vi "TCP_comms_test_receive.vi"() -> ()   [LabVIEW 2018]
panel:
  out "connection ID":refnum<k5>
  in  "Open Connection":bool
  in  "address":string="192.168.0.34"
  out "Received value/i":u32
  out "Connection opened?":bool
  out "Error Out":errorcluster
  in  "Stop and Exit":bool
  in  "Error In":errorcluster
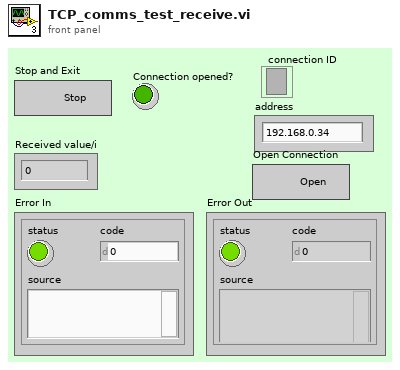
[diagram p1: front panel]
types:
  T1 = enum16{"Standard", "Buffered", "CRLF", "Immediate"}
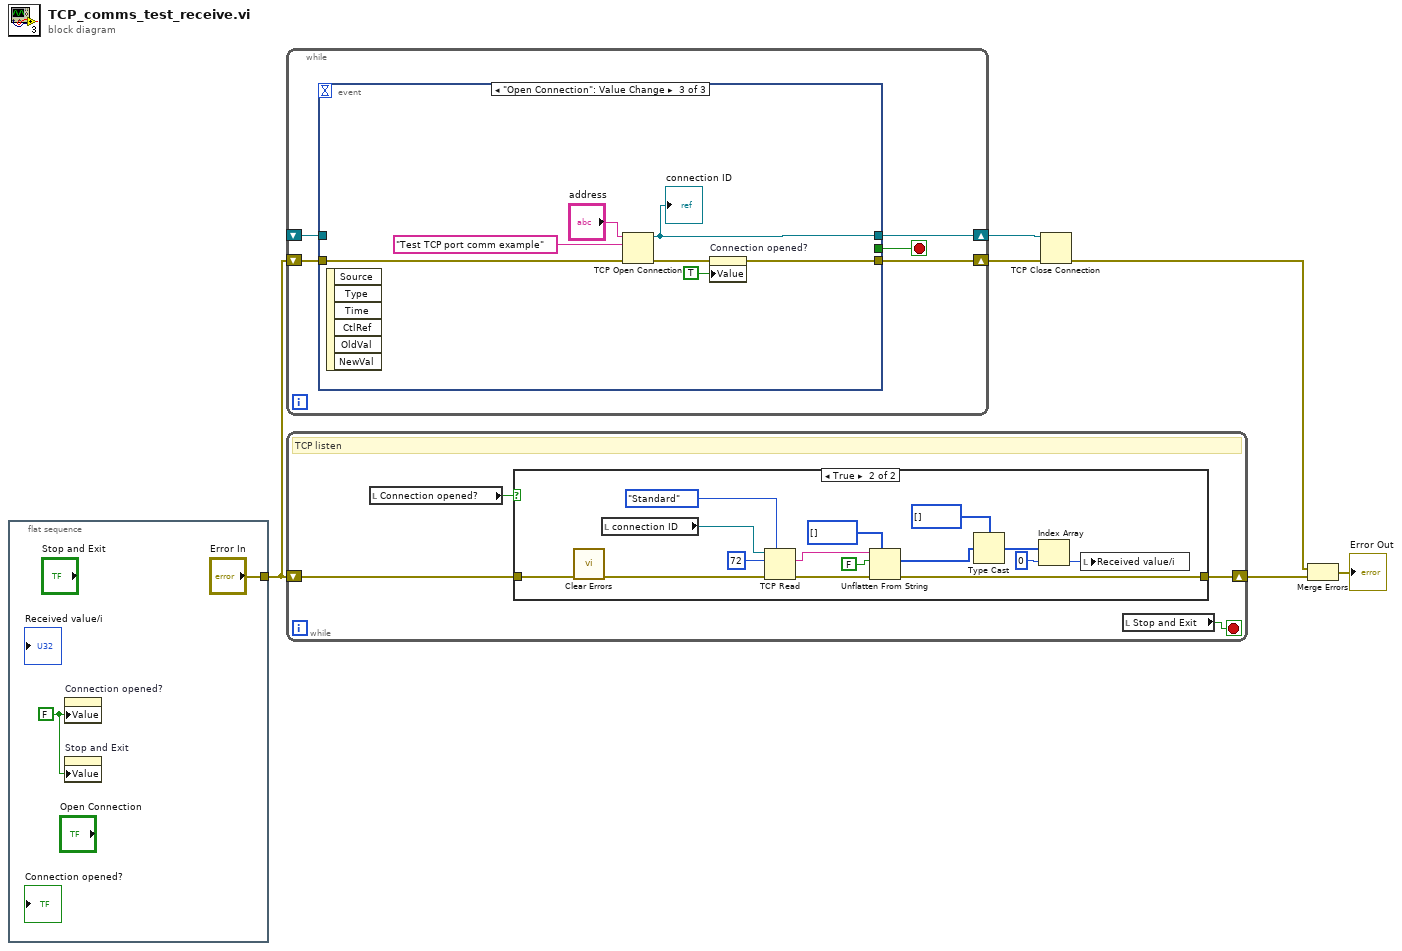
[diagram p0: block diagram]
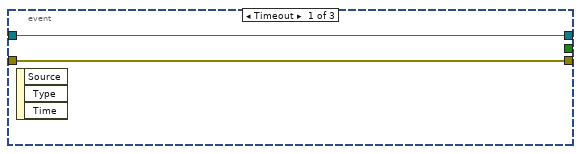
[diagram p3: hidden frame]
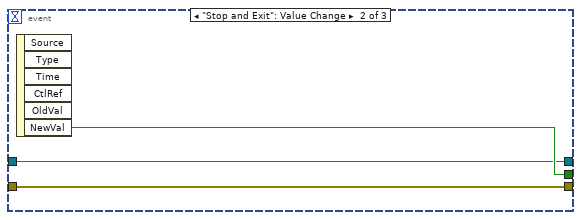
[diagram p4: hidden frame]
diagram:
  n1 = flat-sequence {
    tunnel: ["Error In"] -> w6
    frame #0 {
      w7 = FALSE ("Stop and Exit")
      n2 = property on="Connection opened?" class="Bool (strict)"("Value"=w7) -> ()  [unwired: 2 in, 2 out]
      n3 = property on="Stop and Exit" class="Bool (strict)"("Value"=w7) -> ()  [unwired: 2 in, 2 out]
    }
  }
  n4 = while {
    shift-right: [w11] -> w4
    shift-left: w6 -> [w12]
    shift-right: [w10] -> w1
    shift-left: _ -> [w9]
    stop <- w13 stop-if-true
    n5 = event shown="[2] \"Open Connection\": Value Change" {
      selector: _ -> [_ _ _]
      dyn-events: _ -> [_ _ _]
      timeout: _ -> [_ _ _]
      tunnel: [_ w18 _] -> w13
      tunnel: w12 -> [w15 w17 w25]
      tunnel: [w15 w17 w21] -> w11
      tunnel: [w14 w16 w19] -> w10
      tunnel: w9 -> [w14 w16 _]
      event Timeout {
        n6 = event-data() -> ()  [unwired: 1 in, 3 out]
      }
      event "Stop and Exit": Value Change {
        n7 = event-data() -> ("NewVal"=w18:bool)  [unwired: 1 in, 5 out]
      }
      event "Open Connection": Value Change {
        n8 = event-data() -> ()  [unwired: 1 in, 6 out]
        n9 = TCP Open Connection(address="address", remote port or service name="Test TCP port comm example" ("service name"), error in (no error)=w25) -> (connection ID=w19:refnum<k5>, error out=w22:errorcluster)  [unwired: 2 in]
        "connection ID" <- w19
        n10 = property on="Connection opened?" class="Bool (strict)"(error in=w22, "Value"=TRUE) -> (error out=w21:errorcluster)  [unwired: 1 in, 1 out]
      }
    }
  }
  n11 = while {
    shift-right: [w27] -> w3
    shift-left: w6 -> [w28]
    stop <- w29 stop-if-true
    # "TCP listen"
    n12 = local read "Connection opened?"() -> (w26:bool)
    n13 = case shown="True" w26 {
      tunnel: w28 -> [w30 w37]
      tunnel: [w30 w35] -> w27
      frame False {
      }
      frame True {
        n14 = call <vilib>:"Clear Errors.vi"("error in (no error)"=w37) -> ("error out"=w45:errorcluster)  [unwired: 5 in, 1 out]
        n15 = local read "connection ID"() -> (w31:refnum<k5>)
        n16 = TCP Read(connection ID=w31, bytes to read=72, error in (no error)=w45, 7:T1."Standard" ("mode (standard)")) -> (data out=w44:string, error out=w43:errorcluster)  [unwired: 1 in, 1 out]
        n17 = Unflatten From String(type=u8[] [], binary string=w44, data includes array or string size? (T)=FALSE, error in (no error)=w43) -> (value=w40:u8[], error out=w35:errorcluster)  [unwired: 1 in, 1 out]
        n18 = Type Cast(type=u32[] [] ("*(type *) &x"), x=w40) -> (*(type *) &x=w41:u32[])
        n19 = Index Array(array=w41, index=0) -> (element=w33:u32)
        n20 = local write "Received value/i"(w33) -> ()
      }
    }
    n21 = local read "Stop and Exit"() -> (w29:bool)
  }
  n22 = TCP Close Connection(connection ID=w1, error in (no error)=w4) -> (error out=w2:errorcluster)  [unwired: 1 in, 1 out]
  n23 = Merge Errors(w2, w3) -> (→"Error Out":errorcluster)
